vi "Get Base Path.vi"(8 "error in (no error)":errorcluster, 11 "Log File Specification in":refnum<class "Log File Specification.lvclass">) -> (0 "error out":errorcluster, 2 "Base Path":path, 3 "Log File Specification out":refnum<class "Log File Specification.lvclass">)   [LabVIEW 2012, in "Waveform Data Logger Shared.lvlib" / "Log File Specification.lvclass"]
doc: "Gets the base path for the log file, which is used to construct instance file paths based on the specified path tag values when the instance file is opened."
uses:
  Log File Specification.lvclass
  Log File Specification.lvclass/Log File Specification.ctl
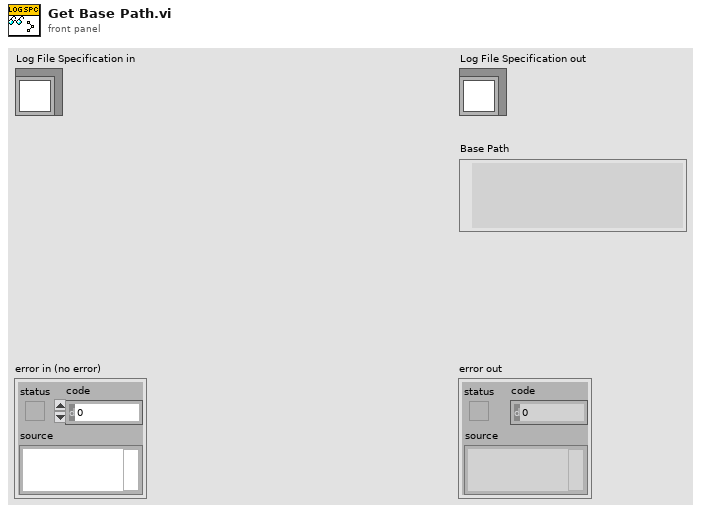
[diagram p1: front panel]
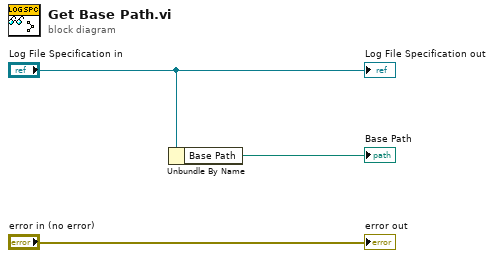
[diagram p0: block diagram]
diagram:
  n1 = Unbundle By Name("Log File Specification in") -> ("Base Path"=→"Base Path":path)
  "error out" <- "error in (no error)"
  "Log File Specification out" <- "Log File Specification in"
